vi "Calibration Offset (Read).vi"(6 "ISOBUS address":T3=-1 caption="ISOBUS address (-1)", 8 "error in":errorcluster, 11 "Mercury Reference In":T4) -> (0 "error out":errorcluster, 2 "Offset Factor":dbl, 3 "Mercury Reference Out":T4, 4 "Valid?":T2)   [LabVIEW 2014, in "Mercury iXX.lvlib" / "Temperature.lvlib"]
doc: "Read the current calibration offset for the selected temperature device."
uses:
  Temperature.lvlib
  Controls/Mercury Reference.ctl
  Controls/Comms Transport Layer.ctl
  Private/Controls/Query Dynamic Reference.ctl
  Controls/ISOBus Address.ctl
  Controls/Is Valid LED.ctl
  Controls/Unit String.ctl
  Private/Controls/Command Verbs.ctl
  Mercury iXX.lvlib
panel:
  out "Unit":T1
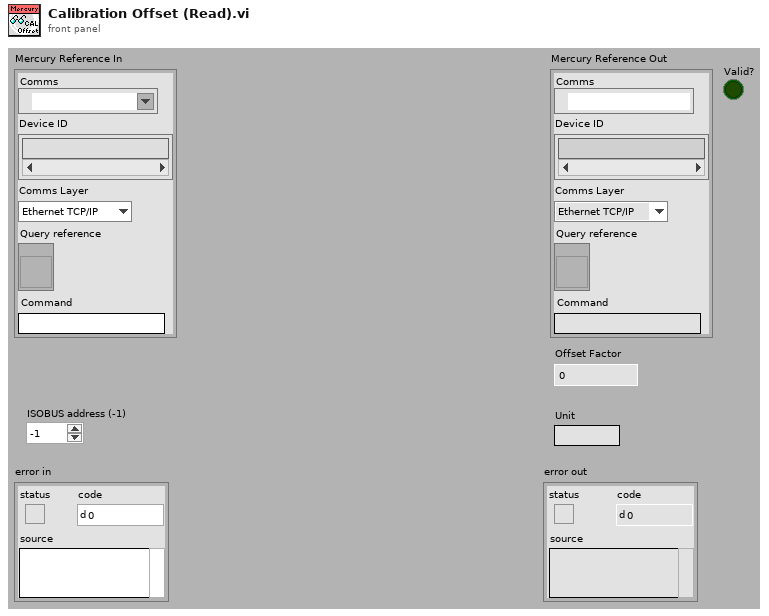
[diagram p1: front panel]
types:
  T1 = typedef "Mercury iXX.lvlib/Unit String.ctl" = string
  T2 = typedef "Mercury iXX.lvlib/Is Valid LED.ctl" = bool
  T3 = typedef "Mercury iXX.lvlib/ISOBus Address.ctl" = i32
  T4 = typedef "Mercury iXX.lvlib/Mercury Reference.ctl" = cluster{"Comms":refnum<visa-resource-name>, "Device ID":string[], "Comms Layer":T5, "Command":string, "Query reference":T6}
  T5 = typedef "Mercury iXX.lvlib/Comms Transport Layer.ctl" = enum16{"Ethernet TCP/IP", "USB", "ISOBus - RS-232", "GPIB"}
  T6 = typedef "Mercury iXX.lvlib/Query Dynamic Reference.ctl" = refnum<vi>
  T7 = typedef "Mercury iXX.lvlib/Command Verbs.ctl" = string
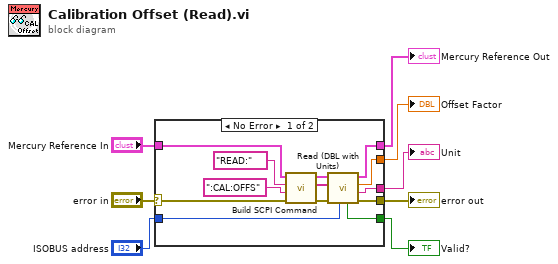
[diagram p0: block diagram]
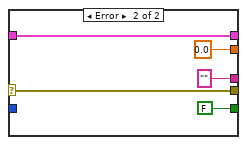
[diagram p2: hidden frame]
diagram:
  n1 = case shown="No Error" "error in" {
    selector: "error in" -> [w10 w25]
    tunnel: "Mercury Reference In" -> [w18 w26]
    tunnel: [w17 w26] -> w7
    tunnel: [w16 w25] -> w6
    tunnel: [w14 0.0 ("Data (Dbl)")] -> w5
    tunnel: [w13 T1 "" ("Unit")] -> w4
    tunnel: [w12 T2 FALSE ("Valid?")] -> w3
    tunnel: "ISOBUS address" -> [w9 _]
    frame No Error {
      n2 = call "Build SCPI Command.vi"("error in"=w10, "Noun(s)"=":CAL:OFFS" ("Command"), "Verb"=T7 "READ:", "Mercury Reference In"=w18) -> ("error out"=w15:errorcluster, "SCPI Message(s)"=w20:string[], "Mercury Reference Out"=w21:T4)  [unwired: 5 out]
      n3 = call "Read (DBL with Units).vi"("ISOBUS address"=w9, "error in"=w15, "SCPI Message(s)"=w20, "Mercury Reference In"=w21) -> ("error out"=w16:errorcluster, "Unit"=w13:T1, "Data (Dbl)"=w14:dbl, "Mercury Reference Out"=w17:T4, "Valid?"=w12:T2)  [unwired: 3 out]
    }
    frame Error {
    }
  }
  "Mercury Reference Out" <- w7
  "error out" <- w6
  "Offset Factor" <- w5
  "Valid?" <- w3
  "Unit" <- w4
